vi "signalgen.vi"() -> ()   [LabVIEW 2020]
uses:
  <vilib>/measure/maspectr.llb/FFT Power Spectrum and PSD for 1 Chan.vi
  <vilib>/measure/NI_MABase.lvlib
  <vilib>/measure/NI_MAPro.lvlib
panel:
  in  "Cluster":cluster{"Sampling Freq":dbl, "Samples":dbl}
  in  "Logarithmic Scale":bool
  in  "Window":u32(ring)=1 items=["Rectangle"=0, "Hanning"=1, "Hamming"=2, "Blackman-Harris"=3, "Exact Blackman"=4, "Blackman"=5, "Flat Top"=6, "4 Term B-Harris "=7, "7 Term B-Harris"=8, "Low Sidelobe"=9, "Blackman Nuttall"=11, "Triangle"=30, "Bartlett-Hanning"=31, "Bohman"=32, "Parzen"=33, "Welch"=34, "Kaiser"=60, "Dolph-Chebyshev"=61, "Gaussian"=62]
  in  "stop":bool
  in  "Signal type":u16(ring) items=["Sine Wave", "Triangle Wave", "Square Wave", "Sawtooth Wave"]
  in  "Signal class":u16(ring) items=["Noise", "Periodic"]
  in  "Czestotliwosc":dbl(knob) scale=0.01..500.0
  in  "Amplituda":dbl(knob) scale=0.01..10.0
  out "Signal Waveform":waveform(dbl)(graph)
  out "Frequency Spectrum":cluster{"f0":dbl, "df":dbl, "magnitude":dbl[]}(graph)
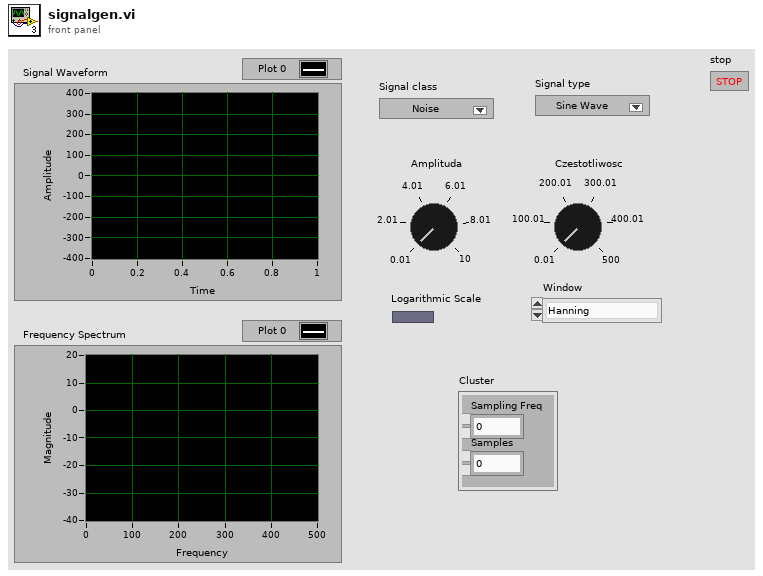
[diagram p1: front panel]
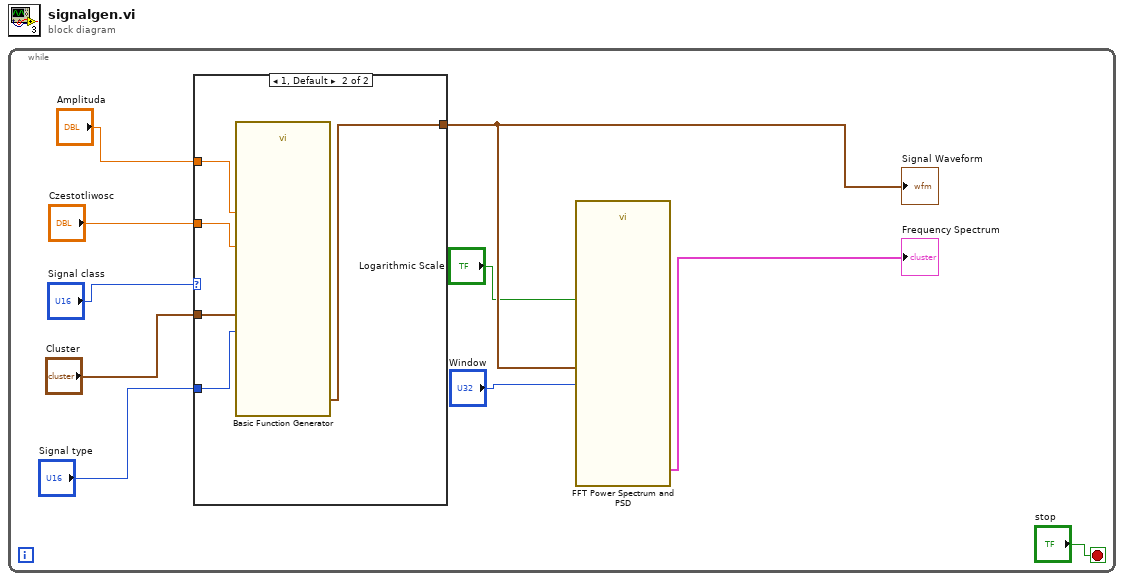
[diagram p0: block diagram]
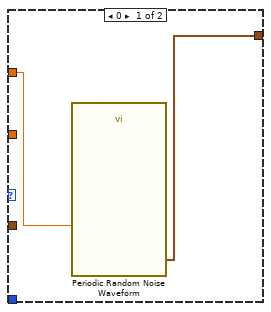
[diagram p2: hidden frame]
diagram:
  n1 = while {
    stop <- "stop" stop-if-true
    n2 = case shown="1, Default" "Signal class" {
      tunnel: "Amplituda" -> [w12 w17]
      tunnel: "Czestotliwosc" -> [_ w16]
      tunnel: "Signal type" -> [_ w15]
      tunnel: [w11 w14] -> w5
      tunnel: "Cluster" -> [_ w13]
      frame 0 {
        n3 = call <vilib>:"Periodic Random Noise Waveform.vi"("spectral amplitude"=w12) -> ("signal out"=w11:waveform(dbl))  [unwired: 9 in, 1 out]
      }
      frame 1, Default {
        n4 = call <vilib>:"Basic Function Generator.vi"("sampling info"=w13, "signal type"=w15, "amplitude"=w17, "frequency"=w16) -> ("signal out"=w14:waveform(dbl))  [unwired: 5 in, 2 out]
      }
    }
    "Signal Waveform" <- w5
    n5 = call-poly <vilib>:"FFT Power Spectrum and PSD.vi"("dB On (F)"="Logarithmic Scale", "window"="Window", "time signal"=w5) -> ("Power Spectrum / PSD"=→"Frequency Spectrum":cluster{"f0":dbl, "df":dbl, "magnitude":dbl[]})  [unwired: 5 in, 3 out]
  }
